vi "KE622x -- Set Trig Layer Params.vi"(0 "Resource In":refnum<visa-resource-name>, 1 "Check For SCPI Errors? (T)":bool=TRUE, 7 "Trig Layer Params In":T1, 11 "error in (no error)":errorcluster, 12 "Read Back Set Values? (T)":bool=TRUE) -> (4 "Resource Out (dupl)":refnum<visa-resource-name>, 8 "Trig Layer Params Out":T1, 15 "error out":errorcluster)   [LabVIEW 2019, in "Keithley 622x.lvlib"]
doc: "Sets the parameters for the 'Trigger' layer of the trigger model."
uses:
  Keithley 622x.lvlib
  Typedefs/KE622x -- Trig Layer Params.ctl
  Low Level/Typedefs/KE622x -- Trig Source.ctl
  Low Level/Typedefs/KE622x -- Trig Link Line.ctl
  Low Level/Typedefs/KE622x -- Trig Output Mode.ctl
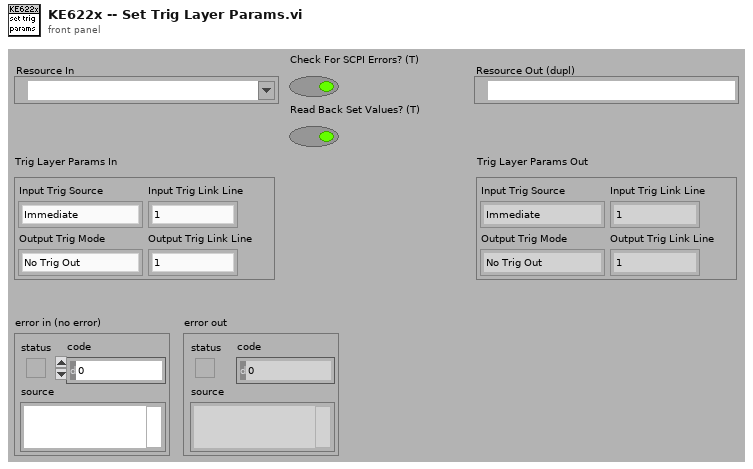
[diagram p1: front panel]
types:
  T1 = typedef "Keithley 622x.lvlib/KE622x -- Trig Layer Params.ctl" = cluster{"Input Trig Source":T2, "Input Trig Link Line":T3, "Output Trig Mode":T4, "Output Trig Link Line":T3}
  T2 = typedef "Keithley 622x.lvlib/KE622x -- Trig Source.ctl" = enum16{"Immediate", "Trigger Link"}
  T3 = typedef "Keithley 622x.lvlib/KE622x -- Trig Link Line.ctl" = enum16{"1", "2", "3", "4", "5", "6"}
  T4 = typedef "Keithley 622x.lvlib/KE622x -- Trig Output Mode.ctl" = enum16{"No Trig Out", "Source Turn On", "After Source Delay"}
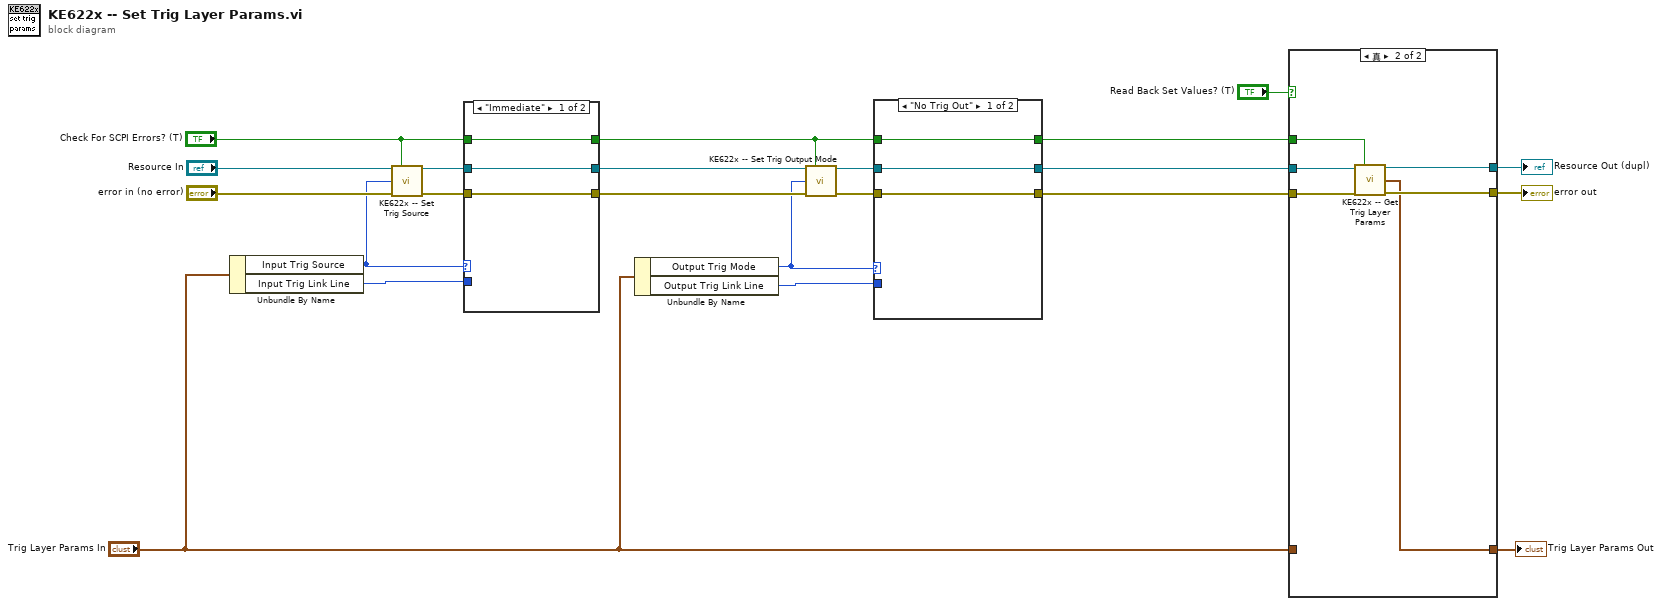
[diagram p0: block diagram]
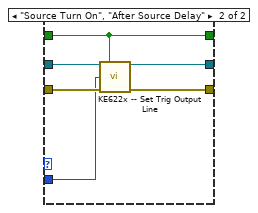
[diagram p2: hidden frame]
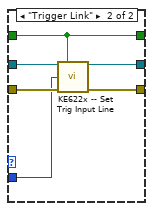
[diagram p3: hidden frame]
diagram:
  n1 = Unbundle By Name("Trig Layer Params In") -> ("Input Trig Source"=w17:T2, "Input Trig Link Line"=w13:T3)
  n2 = call "KE622x -- Set Trig Source.vi"("Resource In"="Resource In", "Check For SCPI Errors? (T)"="Check For SCPI Errors? (T)", "Trig Source"=w17, "error in (no error)"="error in (no error)") -> ("Resource Out (dupl)"=w16:refnum<visa-resource-name>, "error out"=w15:errorcluster)  [unwired: 10 in]
  n3 = case shown="\"Immediate\"" w17 {
    tunnel: w16 -> [w25 w31]
    tunnel: w15 -> [w24 w30]
    tunnel: [w25 w27] -> w11
    tunnel: [w24 w28] -> w10
    tunnel: "Check For SCPI Errors? (T)" -> [w23 w26]
    tunnel: w13 -> [_ w29]
    tunnel: [w23 w26] -> w6
    frame "Immediate" {
    }
    frame "Trigger Link" {
      n4 = call "KE622x -- Set Trig Input Line.vi"("Resource In"=w31, "Check For SCPI Errors? (T)"=w26, "Trig Input Line"=w29, "error in (no error)"=w30) -> ("Resource Out (dupl)"=w27:refnum<visa-resource-name>, "error out"=w28:errorcluster)  [unwired: 10 in]
    }
  }
  n5 = Unbundle By Name("Trig Layer Params In") -> ("Output Trig Mode"=w9:T4, "Output Trig Link Line"=w5:T3)
  n6 = call "KE622x -- Set Trig Output Mode.vi"("Resource In"=w11, "Check For SCPI Errors? (T)"=w6, "Trig Output Mode"=w9, "error in (no error)"=w10) -> ("Resource Out (dupl)"=w8:refnum<visa-resource-name>, "error out"=w7:errorcluster)  [unwired: 10 in]
  n7 = case shown="\"No Trig Out\"" w9 {
    tunnel: w8 -> [w34 w40]
    tunnel: w7 -> [w33 w39]
    tunnel: [w34 w36] -> w4
    tunnel: [w33 w38] -> w3
    tunnel: w6 -> [w32 w35]
    tunnel: w5 -> [_ w37]
    tunnel: [w32 w35] -> w2
    frame "No Trig Out" {
    }
    frame "Source Turn On", "After Source Delay" {
      n8 = call "KE622x -- Set Trig Output Line.vi"("Resource In"=w40, "Check For SCPI Errors? (T)"=w35, "Trig Output Line"=w37, "error in (no error)"=w39) -> ("Resource Out (dupl)"=w36:refnum<visa-resource-name>, "error out"=w38:errorcluster)  [unwired: 10 in]
    }
  }
  n9 = case shown="真" "Read Back Set Values? (T)" {
    tunnel: [w41 w49] -> w20
    tunnel: [w42 w48] -> w21
    tunnel: "Trig Layer Params In" -> [w43 _]
    tunnel: [w43 w47] -> w1
    tunnel: w4 -> [w42 w46]
    tunnel: w3 -> [w41 w45]
    tunnel: w2 -> [_ w44]
    frame False {
    }
    frame True {
      n10 = call "KE622x -- Get Trig Layer Params.vi"("Resource In"=w46, "Check For SCPI Errors? (T)"=w44, "error in (no error)"=w45) -> ("Resource Out (dupl)"=w48:refnum<visa-resource-name>, "Trig Layer Params"=w47:T1, "error out"=w49:errorcluster)  [unwired: 10 in]
    }
  }
  "Resource Out (dupl)" <- w21
  "error out" <- w20
  "Trig Layer Params Out" <- w1
